vi "Core_[HSMS]Selected_Receive Message.vi"(8 "error in (no error)":errorcluster, 10 "Message Packet":T1, 11 "HSMS Class in":refnum<class "HSMS Class.lvclass">) -> (0 "error out":errorcluster, 3 "HSMS Class out":refnum<class "HSMS Class.lvclass">)   [LabVIEW 2020, in "SECS Communication.lvlib" / "HSMS Class.lvclass"]
uses:
  HSMS Class.lvclass
  Message Packet.ctl
  HSMS Class.lvclass/HSMS Class.ctl
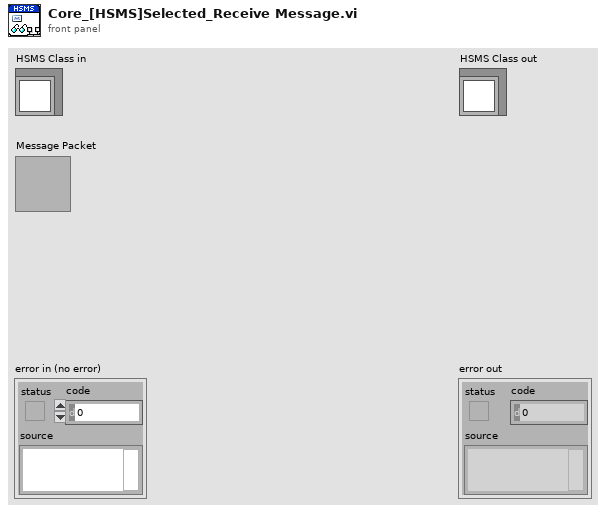
[diagram p1: front panel]
types:
  T1 = typedef "SECS Communication.lvlib/HSMS Class.lvclass/Message Packet.ctl" = cluster{"Message Header Cluster":T2, "Message Header":u8[], "Message Text":u8[]}
  T2 = typedef "SECS Communication.lvlib/HSMS Class.lvclass/Message Header.ctl" = cluster{"Byte 0-1(Session ID)":u16, "W-Bit":bool, "Byte 2":u8, "Byte 3":u8, "Byte 4(PType)":T3, "Byte 5(SType)":T4, "Byte 6-9(System Btyes)":u8[]}
  T3 = typedef "SECS Communication.lvlib/HSMS Class.lvclass/PType.ctl" = enum8{"SECS-II Encoding", "Reserved"}
  T4 = typedef "SECS Communication.lvlib/HSMS Class.lvclass/SType.ctl" = enum8{"Data Message", "Select.req", "Select.rsp", "Deselect.req", "Deselect.rsp", "Linktest.req", "Linktest.rsp", "Reject.req", "Separate.req"}
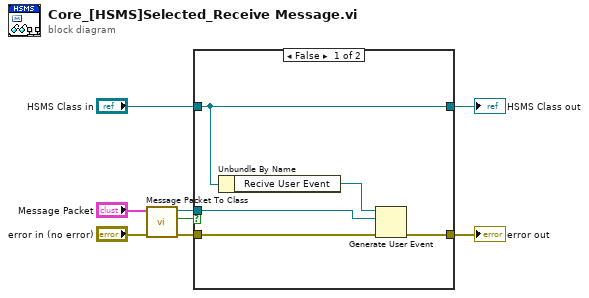
[diagram p0: block diagram]
diagram:
  n1 = call "Message Packet To Class.vi"("error in"="error in (no error)", "Message Packet"="Message Packet") -> ("error out"=w4:errorcluster, "Error?"=w3:bool, "SECS-II Class"=w2:refnum<class "SECS-II Class.lvclass">)  [unwired: 7 in]
  n2 = case shown="False" w3 {
    tunnel: w4 -> [w12 w14]
    tunnel: w2 -> [w10 _]
    tunnel: "HSMS Class in" -> [w13 w15]
    tunnel: [w13 w15] -> w8
    tunnel: [w9 w14] -> w7
    frame False {
      n3 = Unbundle By Name(w13) -> ("Recive User Event"=w11:refnum<user-event>)
      n4 = Generate User Event(user event=w11, event data cluster=w10, error in=w12) -> (error out=w9:errorcluster)  [unwired: 1 in, 1 out]
    }
    frame True {
    }
  }
  "error out" <- w7
  "HSMS Class out" <- w8
